vi "LI-U8 ratio of MSD.vi"(3 "Large number - U8 B":T1, 5 "Large number - U8 A":T1) -> (1 "ratio of MSDs":u8)   [LabVIEW 2012]
doc: "Determines the interger ratio (rounded down) of two LI-U8 format numbers, given that they are within 256 of each other and A is bigger than B"
uses:
  User Access Type defs/Large number - U8 array.ctl
panel:
  # "index 0 = LSD"
  # "always>0"
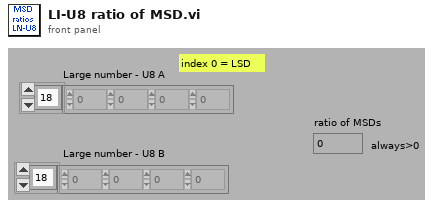
[diagram p1: front panel]
types:
  T1 = typedef "Large number - U8 array.ctl" = u8[]
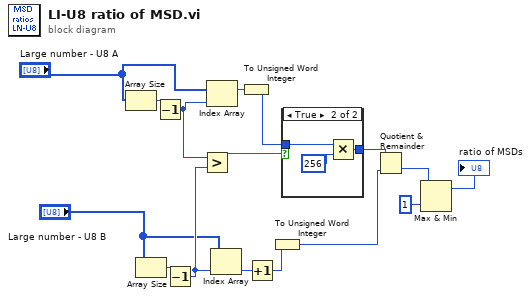
[diagram p0: block diagram]
diagram:
  n1 = Array Size(array="Large number - U8 A") -> (size(s)=w16:i32)
  n2 = Array Size(array="Large number - U8 B") -> (size(s)=w15:i32)
  n3 = Decrement(x=w16) -> (x-1=w14:i32)
  n4 = Decrement(x=w15) -> (x-1=w13:i32)
  n5 = Greater?(x=w14, y=w13) -> (0:w8:bool)
  n6 = Index Array(array="Large number - U8 A", index=w14) -> (element=w12:u8)
  n7 = Index Array(array="Large number - U8 B", index=w13) -> (element=w10:u8)
  n8 = To Unsigned Word Integer(number=w12) -> (unsigned 16bit integer=w11:u16)
  n9 = Increment(x=w10) -> (x+1=w4:u8)
  n10 = To Unsigned Word Integer(number=w4) -> (unsigned 16bit integer=w9:u16)
  n11 = case shown="True" w8 {
    tunnel: w11 -> [w17 w20]
    tunnel: [w17 w18] -> w7
    frame False {
    }
    frame True {
      n12 = Multiply(x=w20, y=u16 256) -> (x*y=w18:u16)
    }
  }
  n13 = Quotient & Remainder(x=w7, y=w9) -> (floor(x/y)=w3:u16)  [unwired: 1 out]
  n14 = Max & Min(x=w3, y=u16 1) -> (max(x,y)=→"ratio of MSDs":u16)  [unwired: 1 out]
